vi "FTP_retrieveConfig.vi"() -> (0 "error out":errorcluster, 3 "local path":path)   [LabVIEW 2014]
uses:
  <vilib>/FTP/NI_FTP.lvlib
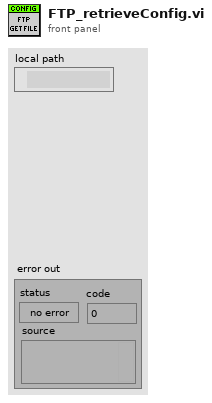
[diagram p1: front panel]
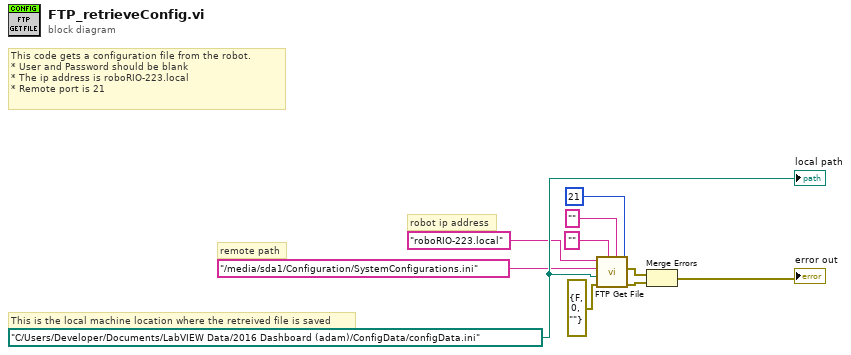
[diagram p0: block diagram]
diagram:
  w9 = path "C:/Users/Developer/Documents/LabVIEW Data/2016 Dashboard (adam)/ConfigData/configData.ini" ("local path")
  # "robot ip address"
  # "remote path"
  # "This is the local machine location where the retreived file is saved"
  # "This code gets a configuration file from the robot. \n* User and Password should be blank            \n* The ip address is roboRIO-223.local\n* Remote port is 21"
  n1 = call <vilib>:"FTP Get File.vi"("remote port (21)"=u16 21, "password"="", "user"="", "error in (no error)"=errorcluster {"status"=FALSE, "code"=0, "source"=""}, "local path"=w9, "remote path"="/media/sda1/Configuration/SystemConfigurations.ini", "host"="roboRIO-223.local") -> ("error out"=w2:errorcluster, "file error"=w3:errorcluster)  [unwired: 3 in]
  n2 = Merge Errors(w3, w2) -> (→"error out":errorcluster)
  "local path" <- w9
